vi "CONTROLES_STRINGS.vi"(11 "vi path":path) -> (0 "error out":errorcluster, 3 "output cluster":cluster{refnum<vi>[]})   [LabVIEW 2019]
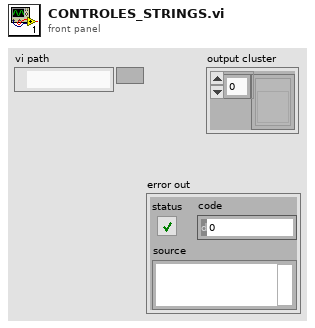
[diagram p1: front panel]
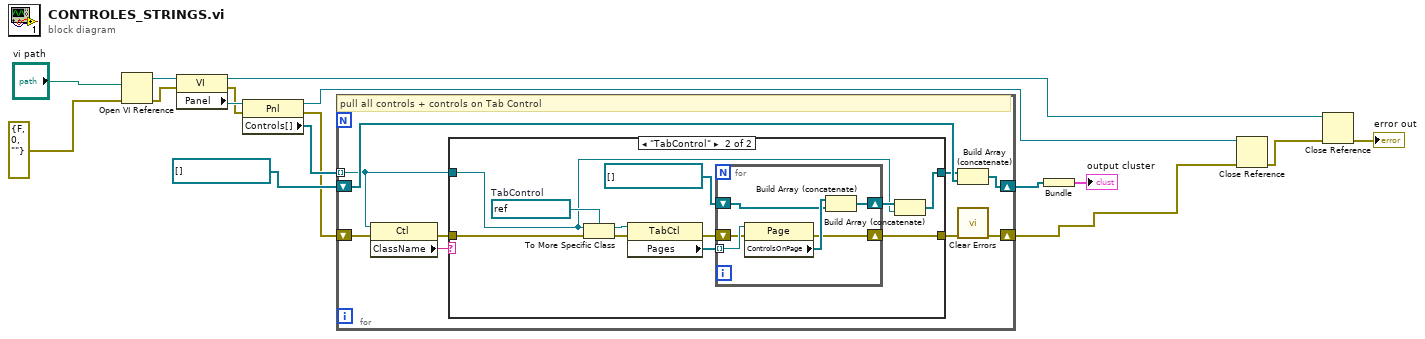
[diagram p0: block diagram]
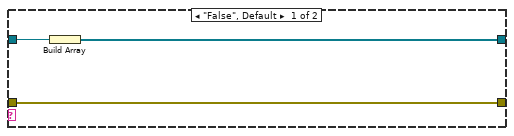
[diagram p2: hidden frame]
diagram:
  n1 = Open VI Reference(vi path="vi path", error in (no error)=errorcluster {"status"=FALSE, "code"=0, "source"=""}) -> (vi reference=w16:refnum<vi>, error out=w9:errorcluster)  [unwired: 4 in]
  n2 = property class="VI"(reference=w16, error in=w9) -> (reference out=w5:refnum<vi>, error out=w8:errorcluster, "Panel"=w15:refnum<vi>)
  n3 = property class="Pnl"(reference=w15, error in=w8) -> (reference out=w1:refnum<vi>, error out=w12:errorcluster, "Controls[]"=w13:refnum<vi>[])
  n4 = for {
    tunnel: w13 -> [w22] mode=indexing
    shift-right: [w23] -> w11
    shift-left: refnum<vi>[] [] -> [w25]
    shift-right: [w19] -> w3
    shift-left: w12 -> [w20]
    # "pull all controls + controls on Tab Control"
    n5 = property class="Ctl"(reference=w22, error in=w20) -> (error out=w18:errorcluster, "ClassName"=w21:string)  [unwired: 1 out]
    n6 = case shown="\"TabControl\"" w21 {
      tunnel: w22 -> [w28 w32]
      tunnel: [w27 w33] -> w24
      tunnel: w18 -> [w26 w31]
      tunnel: [w26 w30] -> w17
      frame "False", Default {
        n7 = Build Array(w28) -> (w27:refnum<vi>[])
      }
      frame "TabControl" {
        w35 = refnum<vi> refnum  # TabControl
        n8 = To More Specific Class(target class=w35, reference=w32, error in=w31) -> (specific class reference=w38:refnum<vi>, error out=w39:errorcluster)
        n9 = property class="TabCtl"(reference=w38, error in=w39) -> (error out=w29:errorcluster, "Pages"=w37:refnum<vi>[])  [unwired: 1 out]
        n10 = for {
          tunnel: w37 -> [w45] mode=indexing
          shift-right: [w44] -> w34
          shift-left: refnum<vi>[] [] ("Controls on Page[]") -> [w42]
          shift-right: [w41] -> w30
          shift-left: w29 -> [w40]
          n11 = property class="Page"(reference=w45, error in=w40) -> (error out=w41:errorcluster, "ControlsOnPage"=w43:refnum<vi>[])  [unwired: 1 out]
          n12 = Build Array (concatenate)(w43, w42) -> (w44:refnum<vi>[])
        }
        n13 = Build Array (concatenate)(w34, w32) -> (w33:refnum<vi>[])
      }
    }
    n14 = Build Array (concatenate)(w24, w25) -> (w23:refnum<vi>[])
    n15 = call <vilib>:"Clear Errors.vi"("error in (no error)"=w17) -> ("error out"=w19:errorcluster)  [unwired: 5 in, 1 out]
  }
  n16 = Bundle(w11) -> (→"output cluster":cluster{refnum<vi>[]})  [unwired: 1 in]
  n17 = Close Reference(reference=w1, error in (no error)=w3) -> (error out=w2:errorcluster)
  n18 = Close Reference(reference=w5, error in (no error)=w2) -> (error out=→"error out":errorcluster)
